vi "button_main_00.vi"() -> ()   [LabVIEW 2023]
panel:
  out "Start_aux":bool
  in  "Start":bool
  in  "Stop Button":bool
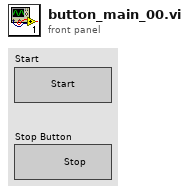
[diagram p1: front panel]
types:
  T1 = enum32{"Bad", "Idle", "Run top level", "Running"}
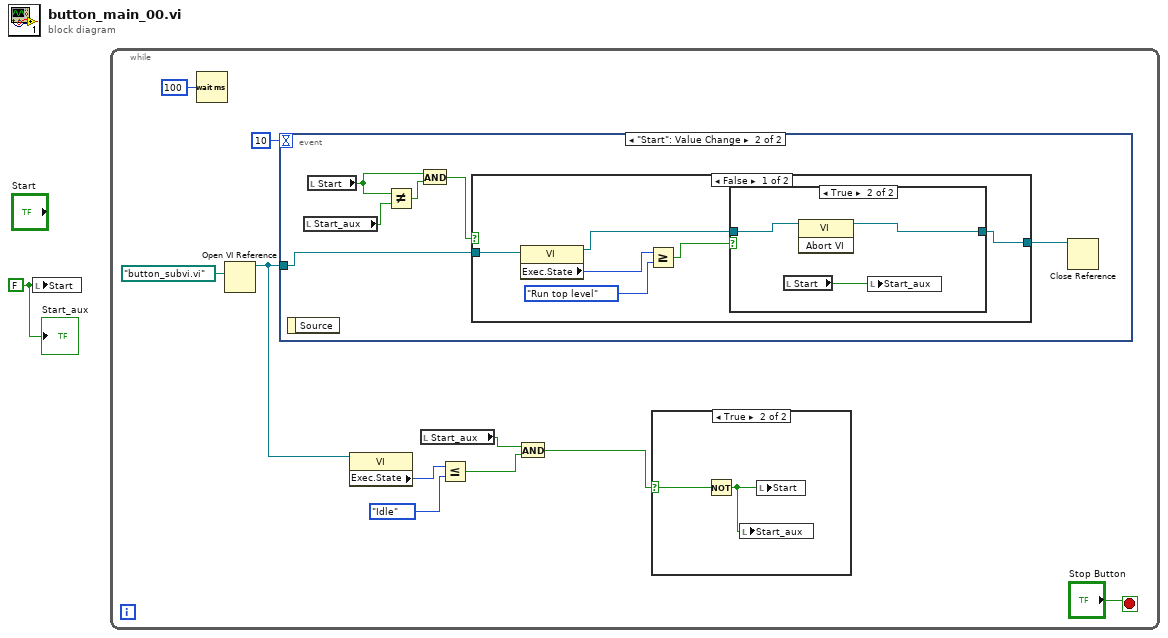
[diagram p0: block diagram]
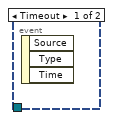
[diagram p3: hidden frame]
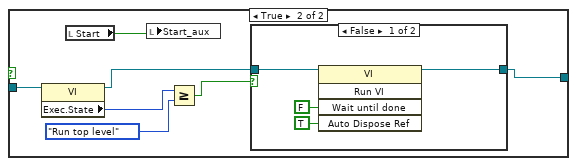
[diagram p5: hidden frame]
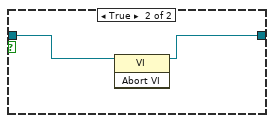
[diagram p6: hidden frame]
diagram:
  w1 = FALSE ("Start")
  n1 = local write "Start"(w1) -> ()
  n2 = while {
    stop <- "Stop Button" stop-if-true
    n3 = Wait (ms)(milliseconds to wait=u32 100) -> ()  [unwired: 1 out]
    n4 = Open VI Reference(vi path=path "button_subvi.vi") -> (vi reference=w7:refnum<vi>)  [unwired: 5 in, 1 out]
    n5 = event shown="[1] \"Start\": Value Change" {
      selector: _ -> [_ _]
      dyn-events: _ -> [_ _]
      timeout: 10 -> [_ _]
      tunnel: w7 -> [_ w19]
      event Timeout {
        n6 = event-data() -> ()  [unwired: 1 in, 3 out]
      }
      event "Start": Value Change {
        n7 = event-data() -> ()  [unwired: 1 in, 1 out]
        n8 = local read "Start_aux"() -> (w17:bool)
        n9 = local read "Start"() -> (w15:bool)
        n10 = Not Equal?(x=w15, y=w17) -> (x != y?=w16:bool)
        n11 = And(x=w15, y=w16) -> (x .and. y?=w14:bool)
        n12 = case shown="False" w14 {
          tunnel: w19 -> [w21 w36]
          tunnel: [w20 w30] -> w18
          frame False {
            n13 = property class="VI"(reference=w21) -> (reference out=w23:refnum<vi>, "Exec.State"=w25:T1)  [unwired: 1 in, 1 out]
            n14 = Greater Or Equal?(x=w25, y=T1."Run top level" ("Execution:State")) -> (x >= y?=w24:bool)
            n15 = case shown="True" w24 {
              tunnel: w23 -> [w26 w29]
              tunnel: [w26 w28] -> w20
              frame False {
              }
              frame True {
                n16 = local read "Start"() -> (w27:bool)
                n17 = invoke class="VI" method="Abort VI"(reference=w29) -> (reference out=w28:refnum<vi>)  [unwired: 2 in, 2 out]
                n18 = local write "Start_aux"(w27) -> ()
              }
            }
          }
          frame True {
            n19 = property class="VI"(reference=w36) -> (reference out=w32:refnum<vi>, "Exec.State"=w34:T1)  [unwired: 1 in, 1 out]
            n20 = local read "Start"() -> (w31:bool)
            n21 = local write "Start_aux"(w31) -> ()
            n22 = Greater Or Equal?(x=w34, y=T1."Run top level" ("Execution:State")) -> (x >= y?=w33:bool)
            n23 = case shown="False" w33 {
              tunnel: w32 -> [w38 w42]
              tunnel: [w37 w41] -> w30
              frame False {
                n24 = invoke class="VI" method="Run VI"(reference=w38, "Wait until done"=FALSE ("Wait Until Done"), "Auto Dispose Ref"=TRUE ("Auto Dispose Reference")) -> (reference out=w37:refnum<vi>)  [unwired: 2 in, 4 out]
              }
              frame True {
                n25 = invoke class="VI" method="Abort VI"(reference=w42) -> (reference out=w41:refnum<vi>)  [unwired: 2 in, 2 out]
              }
            }
          }
        }
        n26 = Close Reference(reference=w18) -> ()  [unwired: 1 in, 1 out]
      }
    }
    n27 = property class="VI"(reference=w7) -> ("Exec.State"=w6:T1)  [unwired: 1 in, 2 out]
    n28 = local read "Start_aux"() -> (w2:bool)
    n29 = Less Or Equal?(x=w6, y=T1."Idle" ("Execution:State")) -> (x <= y?=w4:bool)
    n30 = And(x=w2, y=w4) -> (x .and. y?=w3:bool)
    n31 = case shown="True" w3 {
      selector: w3 -> [_ w13]
      frame False {
      }
      frame True {
        n32 = Not(x=w13) -> (.not. x?=w12:bool)
        n33 = local write "Start_aux"(w12) -> ()
        n34 = local write "Start"(w12) -> ()
      }
    }
  }
  "Start_aux" <- w1
